vi "mclb_init.vi"(8 "error in (no error)":errorcluster, 10 "min size (36, 36)":cluster{"Width":u32, "Height":u32}={"Width"=36, "Height"=36}, 11 "mclb in":refnum<vi>) -> (0 "error out":errorcluster, 2 "default font":T1, 3 "mclb out":refnum<vi>)   [LabVIEW 2017, in "rywindow.lvclass"]
uses:
  rywindow.lvclass
  <vilib>/Utility/miscctls.llb/LVFontTypeDef.ctl
  <vilib>/Utility/miscctls.llb/LVRowAndColumnUnsignedTypeDef.ctl
  <vilib>/Utility/miscctls.llb/LVRowAndColumnTypeDef.ctl
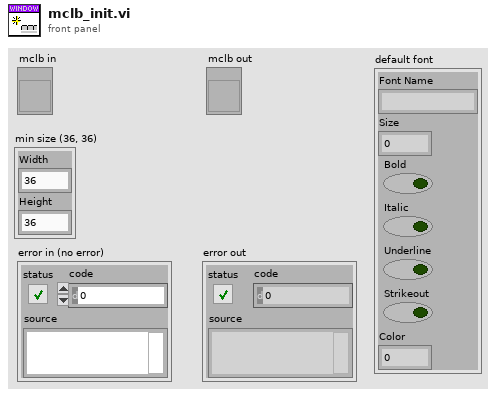
[diagram p1: front panel]
types:
  T1 = typedef "LVFontTypeDef.ctl" = cluster{"Font Name":string, "Size":u16, "Bold":bool, "Italic":bool, "Underline":bool, "Strikeout":bool, "Color":u32}
  T2 = typedef "LVRowAndColumnTypeDef.ctl" = cluster{"Row":i32, "Column":i32}
  T3 = typedef "LVRowAndColumnUnsignedTypeDef.ctl" = cluster{"Row":u32, "Column":u32}
  T4 = typedef "LVRectTypeDef.ctl" = cluster{"Left":i16, "Top":i16, "Right":i16, "Bottom":i16}
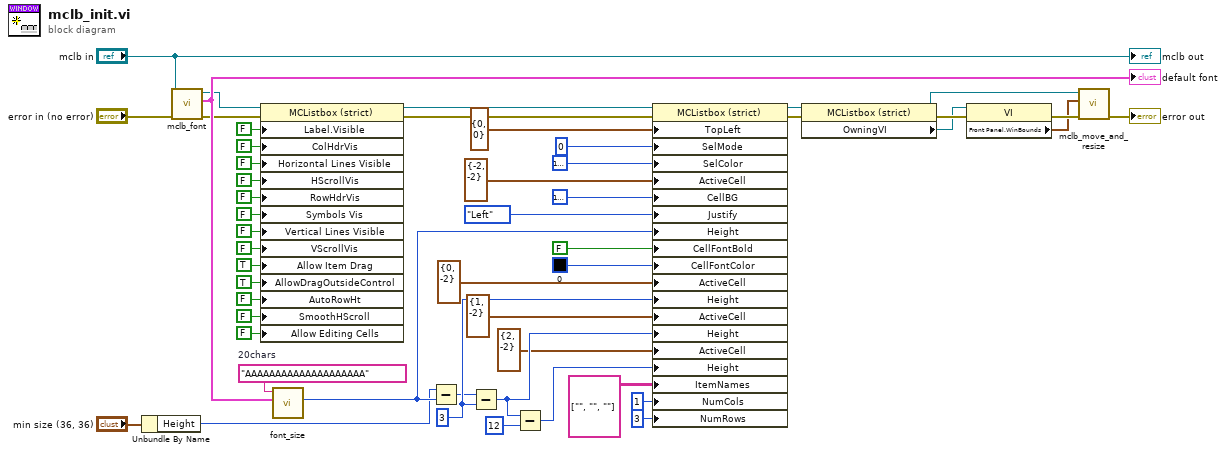
[diagram p0: block diagram]
diagram:
  w39 = "AAAAAAAAAAAAAAAAAAAA"  # 20chars
  w46 = u32 3 ("Active Cell:Cell Size:Height")
  n1 = Unbundle By Name("min size (36, 36)") -> ("Height"=w43:u32)
  n2 = call "mclb_font.vi"("error in (no error)"="error in (no error)", "mclb in"="mclb in") -> ("error out"=w16:errorcluster, "default font"=w49:T1, "mclb out"=w15:refnum<vi>)  [unwired: 7 in]
  "default font" <- w49
  n3 = property class="MCListbox (strict)"(reference=w15, error in=w16, "Label.Visible"=FALSE, "ColHdrVis"=FALSE ("Visible Items:Column Headers Visible"), "Horizontal Lines Visible"=FALSE ("Visible Items:Horizontal Lines Visible"), "HScrollVis"=FALSE ("Visible Items:Horizontal Scrollbar Visible"), "RowHdrVis"=FALSE ("Visible Items:Row Headers Visible"), "Symbols Vis"=FALSE ("Visible Items:Symbols Visible"), "Vertical Lines Visible"=FALSE ("Visible Items:Vertical Lines Visible"), "VScrollVis"=FALSE ("Visible Items:Vertical Scrollbar Visible"), "Allow Item Drag"=TRUE ("Drag/Drop:Allow Dragging"), "AllowDragOutsideControl"=TRUE ("Drag/Drop:Allow Drag and Drop Outside Control"), "AutoRowHt"=FALSE ("Autosizing Row Height"), "SmoothHScroll"=FALSE ("Smooth Horizontal Scrolling"), "Allow Editing Cells"=FALSE) -> (reference out=w30:refnum<vi>, error out=w17:errorcluster)
  n4 = call "font_size.vi"("cell font"=w49, "text"=w39) -> ("height"=w44:u32)  [unwired: 8 in, 1 out]
  n5 = Subtract(x=w43, y=w44) -> (x-y=w45:u32)
  n6 = Subtract(x=w45, y=w46) -> (x-y=w13:u32)
  n7 = Subtract(x=w13, y=u32 12) -> (x-y=w11:u32)
  n8 = property class="MCListbox (strict)"(reference=w30, error in=w17, "TopLeft"=T3 {"Row"=0, "Column"=0} ("Top Left Visible Cell"), "SelMode"=0 ("Selection Mode"), "SelColor"=u32 16777238, "ActiveCell"=T2 {"Row"=-2, "Column"=-2} ("Active Cell:Active Cell"), "CellBG"=u32 16777216, "Justify"=enum16{"Left", "Center", "Right"}."Left" ("Active Cell:Cell Justification"), "Height"=w44, "CellFontBold"=FALSE ("Active Cell:Cell Font:Bold"), "CellFontColor"=u32 0, "ActiveCell"=T2 {"Row"=0, "Column"=-2} ("Active Cell:Active Cell"), "Height"=w46, "ActiveCell"=T2 {"Row"=1, "Column"=-2} ("Active Cell:Active Cell"), "Height"=w13, "ActiveCell"=T2 {"Row"=2, "Column"=-2} ("Active Cell:Active Cell"), "Height"=w11, "ItemNames"=string[][] [[""], [""], [""]] ("Item Names"), "NumCols"=u32 1 ("Number of Columns"), "NumRows"=u32 3 ("Number of Rows")) -> (reference out=w5:refnum<vi>, error out=w9:errorcluster)
  n9 = property class="MCListbox (strict)"(reference=w5, error in=w9) -> (reference out=w1:refnum<vi>, error out=w6:errorcluster, "OwningVI"=w3:refnum<vi>)
  n10 = property class="VI"(reference=w3, error in=w6) -> (error out=w4:errorcluster, "Front Panel.WinBounds"=w2:T4)  [unwired: 1 out]
  n11 = call "mclb_move_and_resize.vi"("error in (no error)"=w4, "Panel Resize.NewBnds"=w2, "mclb in"=w1) -> ("error out"=→"error out":errorcluster)  [unwired: 7 in, 1 out]
  "mclb out" <- "mclb in"
